vi "SSC DCPower Configure Sense with Abort and Init.vi"(0 "DCPower SSC in":T2[](array[typedef]), 5 "Sense":T1=1008 items=["Local"=1008, "Remote"=1009], 11 "error in":errorcluster) -> (4 "DCPower SSC out":T2[](array[typedef]), 15 "error out":errorcluster)   [LabVIEW 2019]
doc: "This VI configures local or remote sense for the sessions."
uses:
  SSC DCPower.ctl
  <instrlib>/niDCPower/nidcpower.llb/niDCPower Sense.ctl
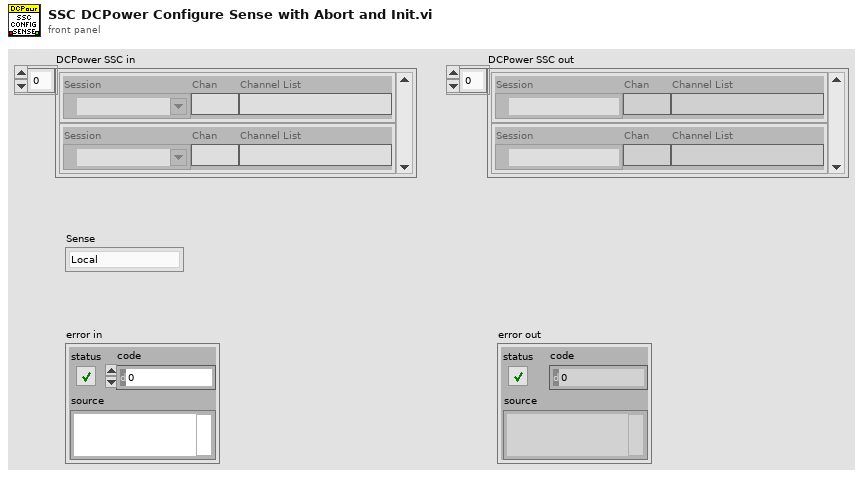
[diagram p1: front panel]
types:
  T1 = typedef "niDCPower Sense.ctl" = i32
  T2 = typedef "SSC DCPower.ctl" = cluster{"Session":refnum<k15>, "Chan":string, "Channel List":string}
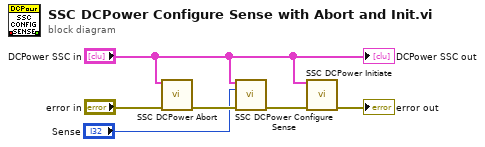
[diagram p0: block diagram]
diagram:
  n1 = call "SSC DCPower Abort.vi"("DCPower SSC in"="DCPower SSC in", "error in"="error in") -> ("error out"=w5:errorcluster)  [unwired: 12 in, 1 out]
  n2 = call "SSC DCPower Configure Sense.vi"("DCPower SSC in"="DCPower SSC in", "Sense"="Sense", "error in"=w5) -> ("error out"=w4:errorcluster)  [unwired: 11 in, 1 out]
  n3 = call "SSC DCPower Initiate.vi"("DCPower SSC in"="DCPower SSC in", "error in"=w4) -> ("error out"=→"error out":errorcluster)  [unwired: 12 in, 1 out]
  "DCPower SSC out" <- "DCPower SSC in"
